vi "test_hardwareactor.vi"() -> ()   [LabVIEW 2015]
panel:
  in  "error in (no error)":errorcluster
  in  "Still Available":bool
  in  "Available":bool
  in  "nr init":i32
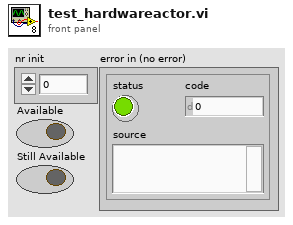
[diagram p1: front panel]
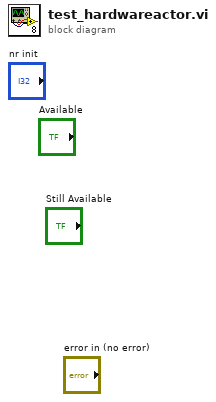
[diagram p0: block diagram]
diagram:
